vi "Friedman2.vi"(8 "error in (no error)":errorcluster caption="entrée d'erreur (pas d'erreur)", 11 "make_friedman2":T2={"n_samples"=100, "noise"=0.0, "random_state"=-1, "Returns"="X"} {"random_state" min=-1; "n_samples" min=1}) -> (0 "error out":errorcluster, 3 "Data":T1)   [LabVIEW 2020]
doc: "Generate the “Friedman #2” regression problem : \n\nThis dataset is described in Friedman1.\n\nInputs X are 4 independent features uniformly distributed on the intervals:\n\n0 <= X[:, 0] <= 100,\n40 * pi <= X[:, 1] <= 560 * pi,\n0 <= X[:, 2] <= 1,\n1 <= X[:, 3] <= 11.\n\nThe output y is created according to the formula:\n\ny(X) = (X[:, 0] ** 2 + (X[:, 1] * X[:, 2] - 1 / (X[:, 1] * X[:, 3])) ** 2) ** 0.5 + noise * N(0, 1).\n\n\n\nParameters : \n\n- n_samples : int, optional (default=100)\nThe number of samples.\n\n- noise : float, optional (default=0.0)\nThe standard deviation of the gaussian noise applied to the output.\n\n- random_state : int, RandomState instance, default=None=-1\nDetermines random number generation for dataset noise. Pass an int for reproducible output across multiple function calls. See Glossary.\n\nReturns : \n\n- X : array of shape [n_samples, 4]\nThe input samples.\n\n- y : array of shape [n_samples]\nThe output values."
uses:
  Friedman2.lvclass
panel:
  out "Friedman2.lvclass":refnum<class "Friedman2.lvclass">
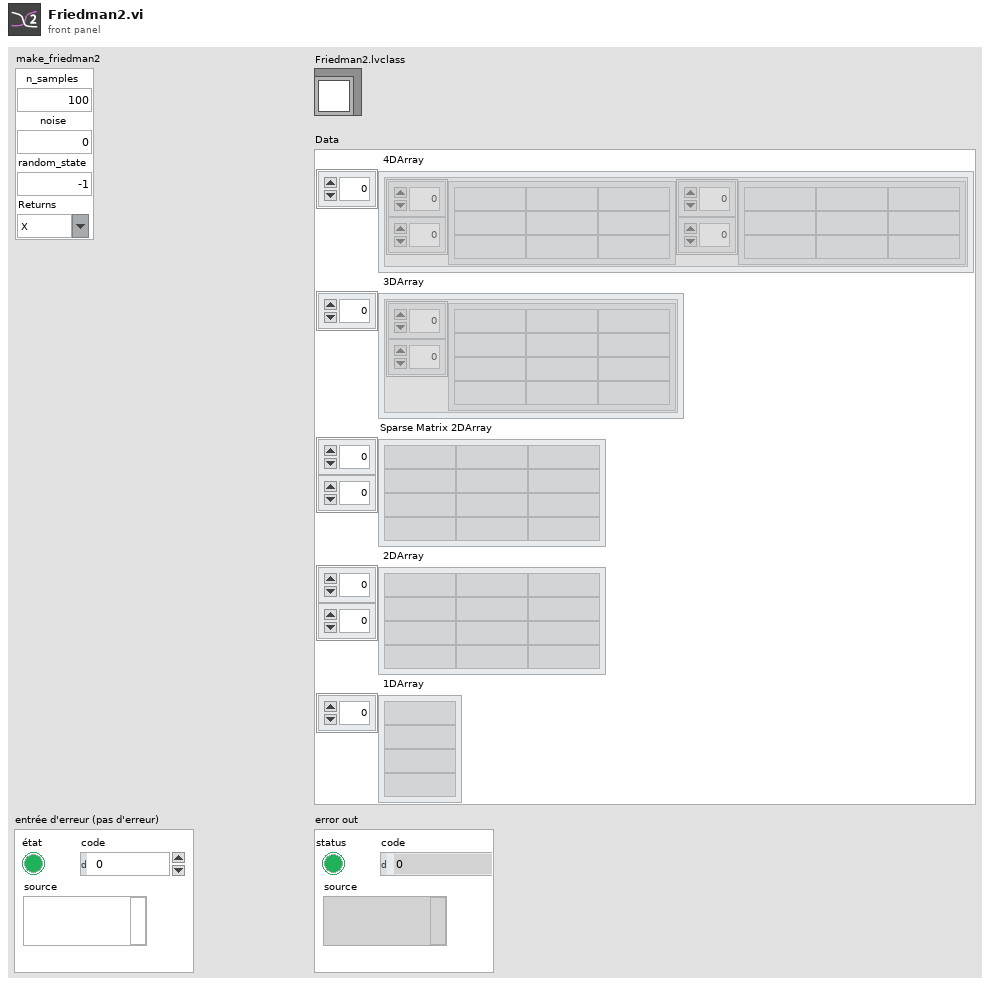
[diagram p1: front panel]
types:
  T1 = cluster{" 4DArray":cluster{"1":string[][], "2":string[][]}[], " 3DArray":cluster{"Tableau":string[][]}[], "Sparse Matrix 2DArray":string[][], " 2DArray":string[][], " 1DArray":string[]}
  T2 = cluster{"n_samples":u32, "noise":dbl, "random_state":i32, "Returns":string}
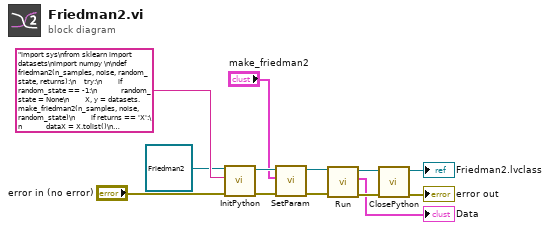
[diagram p0: block diagram]
diagram:
  n1 = call-dynamic "InitPython.vi"("error in (no error)"="error in (no error)", "Python Instruction"="import sys\nfrom sklearn import datasets\nimport numpy \n\ndef friedman2(n_samples, noise, random_state, returns):\n    try:\n        if random_state == -1:\n            random_state = None\n        X, y = datasets.make_friedman2(n_samples, noise, random_state)\n        if returns == 'X':\n            dataX = X.tolist()\n            return str(dataX)\n        else :\n            datay = y.tolist()\n            return str(datay)\n    except:\n        erreur = sys.exc_info()\n        typerr = u\"%s\" % (erreur[0])\n        typerr = typerr[typerr.find(\"'\")+1:typerr.rfind(\"'\")]\n        msgerr = u\"%s\" % (erreur[1])\n        message = str('/!\\\\ {0} : {1}'. format(typerr,msgerr))\n        return message", "Scikit-learn en entrée"=refnum<class "Friedman2.lvclass"> refnum ("Friedman2.lvclass")) -> ("error out"=w8:errorcluster, "Scikit-learn en sortie"=w10:refnum<class "Friedman2.lvclass">)  [unwired: 7 in]
  n2 = call-dynamic "SetParam.vi"("error in (no error)"=w8, "make_friedman2"="make_friedman2", "Friedman2.lvclass"=w10) -> ("error out"=w6:errorcluster, "Friedman2.lvclass"=w7:refnum<class "Friedman2.lvclass">)  [unwired: 7 in]
  n3 = call-dynamic "Run.vi"("error in (no error)"=w6, "Friedman2.lvclass"=w7) -> ("error out"=w4:errorcluster, "Data"=→"Data":T1, "Friedman2.lvclass"=w5:refnum<class "Friedman2.lvclass">)  [unwired: 7 in]
  n4 = call-dynamic "ClosePython.vi"("error in (no error)"=w4, "Scikit-learn en entrée"=w5) -> ("error out"=→"error out":errorcluster, "Scikit-learn en sortie"=→"Friedman2.lvclass":refnum<class "Friedman2.lvclass">)  [unwired: 8 in]
